vi "4Pi 4Pi Modes - Select Modes2.vi"() -> ()   [LabVIEW 2016]
uses:
  4Pi 4Pi Modes - Controls/4Pi 4Pi Modes - Mirror Modes.ctl
  <vilib>/Utility/miscctls.llb/LVPointTypeDef.ctl
  Hardware Configuration/Hardware Configuration Controls/Standard Action.ctl
  4Pi 4Pi Modes - Controls/4Pi 4Pi Modes - Standard Action.ctl
  <userlib>/BMC/BMC.lvlib
panel:
  out "error out":errorcluster
  in  "Mirror Modes":T1
  in  "Flags":string
  in  "Run":bool
  in  "Help":bool
  in  "Control mode":string(combo)="Single"
  in  "DM index":string(combo)="0"
  out "standard output":string
  out "standard error":string
  in  "Calling VI Ref":refnum<vi>
  in  "Exit":bool
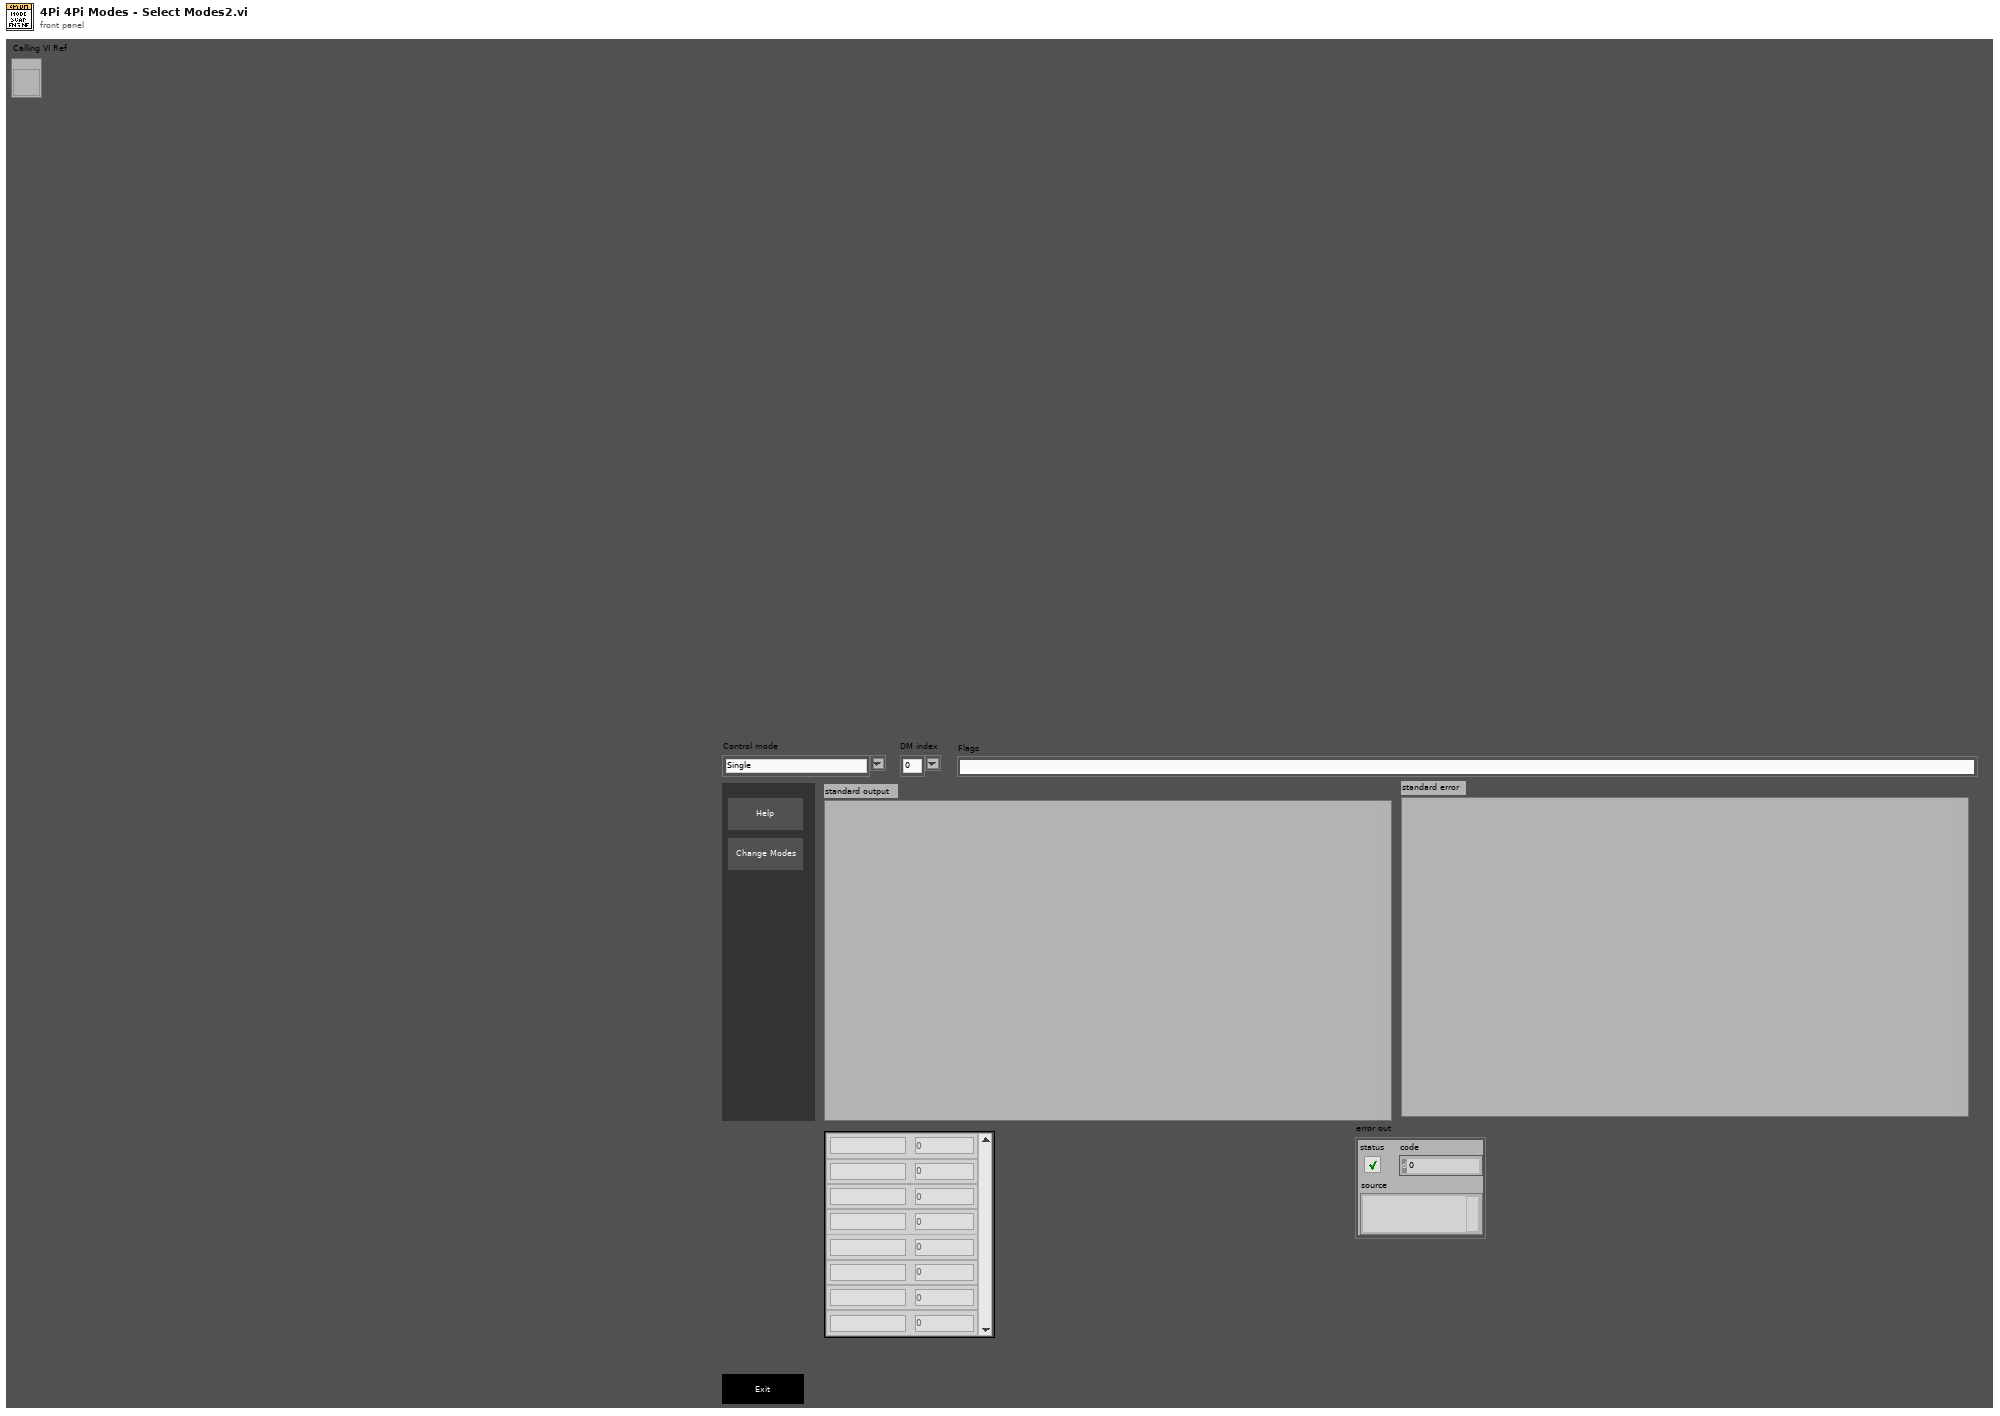
[diagram p1: front panel]
types:
  T1 = typedef "4Pi 4Pi Modes - Mirror Modes.ctl" = cluster{"Mode":string, "Amplitude":dbl}[]
  T2 = enum16{"Always On", "Always Off", "Off While Running"}
  T3 = typedef "LVPointTypeDef.ctl" = cluster{"Horizontal":i16, "Vertical":i16}
  T4 = typedef "LVRectTypeDef.ctl" = cluster{"Left":i16, "Top":i16, "Right":i16, "Bottom":i16}
  T5 = typedef "LVBoundsTypeDef.ctl" = cluster{"Width":u32, "Height":u32}
  T6 = typedef "Standard Action.ctl" = enum16{"Read", "Write"}
  T7 = typedef "4Pi 4Pi Modes - Standard Action.ctl" = enum16{"Read", "Write"}
  T8 = cluster{"type":i16, "ID":i16, "size":i32, "lutName":u64, "priv":u64}[]
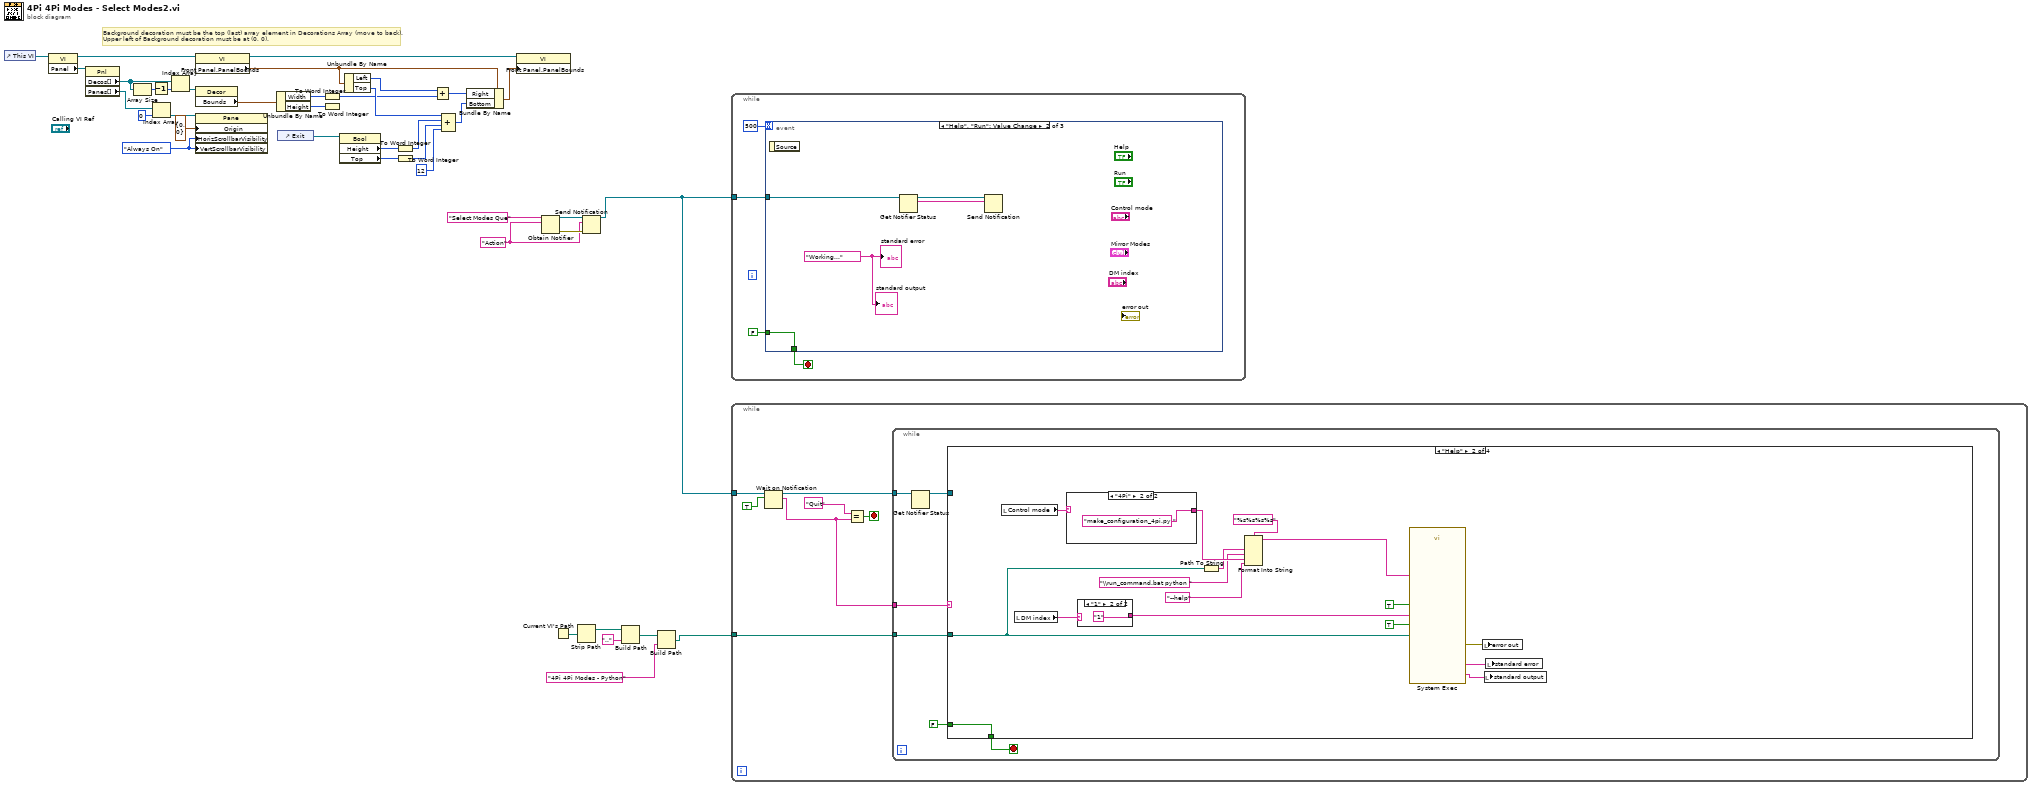
[diagram p0: block diagram]
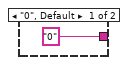
[diagram p3: hidden frame]
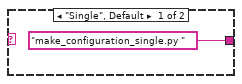
[diagram p4: hidden frame]
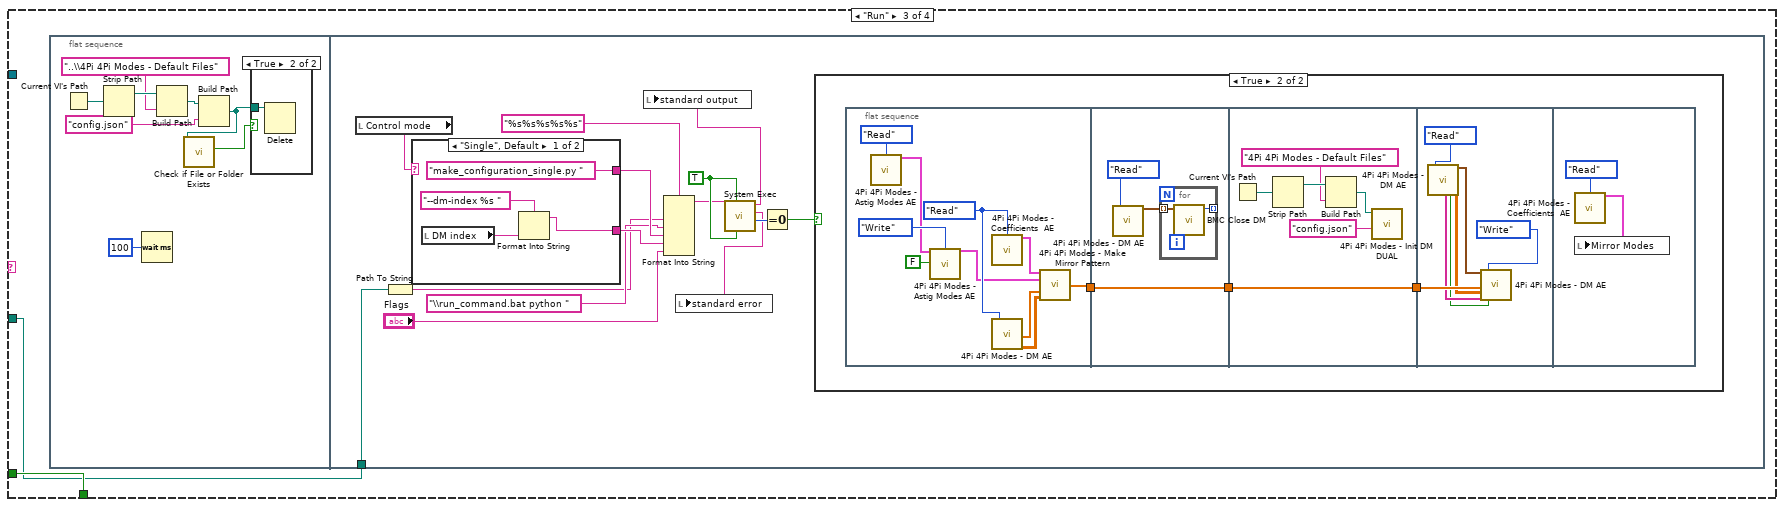
[diagram p5: hidden frame]
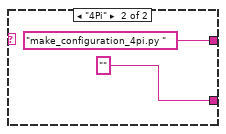
[diagram p8: hidden frame]
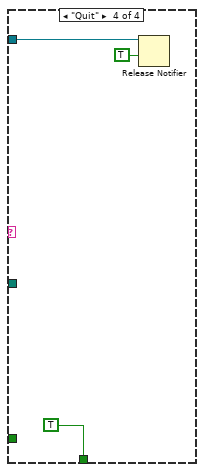
[diagram p9: hidden frame]
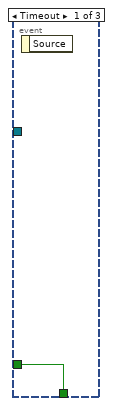
[diagram p10: hidden frame]
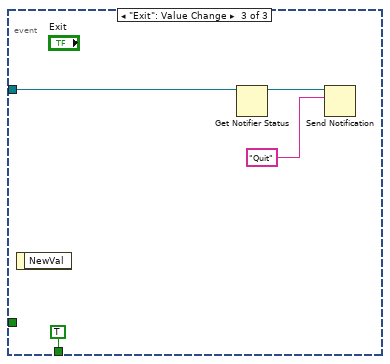
[diagram p11: hidden frame]
diagram:
  w7 = "Action" ("name (unnamed)")
  w23 = T2."Always On" ("Vertical Scrollbar Visibility")
  # "Background decoration must be the top (last) array element in Decorations Array (move to back).\nUpper left of Background decoration must be at (0, 0)."
  n1 = control-ref of="This VI"() -> (w15:refnum<vi>)
  n2 = property class="VI"(reference=w15) -> (reference out=w24:refnum<vi>, "Panel"=w16:refnum<vi>)  [unwired: 1 in, 1 out]
  n3 = property class="Pnl"(reference=w16) -> ("Decos[]"=w14:refnum<vi>[], "Panes[]"=w20:refnum<vi>[])  [unwired: 1 in, 2 out]
  n4 = Array Size(array=w14) -> (size(s)=w12:i32)
  n5 = Decrement(x=w12) -> (x-1=w13:i32)
  n6 = Index Array(array=w20, index=0) -> (element=w19:refnum<vi>)
  n7 = Index Array(array=w14, index=w13) -> (element=w22:refnum<vi>)
  n8 = property class="VI"(reference=w24) -> (reference out=w26:refnum<vi>, "Front Panel.PanelBounds"=w27:T4)  [unwired: 1 in, 1 out]
  n9 = property class="Decor"(reference=w22) -> ("Bounds"=w25:T5)  [unwired: 1 in, 2 out]
  n10 = property class="Pane"(reference=w19, "Origin"=T3 {"Horizontal"=0, "Vertical"=0}, "HorizScrollbarVisibility"=w23, "VertScrollbarVisibility"=w23) -> ()  [unwired: 1 in, 2 out]
  n11 = Unbundle By Name(w25) -> ("Width"=w30:u32, "Height"=w33:u32)
  n12 = control-ref of="Exit"() -> (w17:refnum<vi>)
  n13 = To Word Integer(number=w30) -> (16bit integer=w32:i16)
  n14 = To Word Integer(number=w33) -> ()  [unwired: 1 out]
  n15 = property class="Bool"(reference=w17) -> ("Height"=w35:u32, "Top"=w36:i32)  [unwired: 1 in, 2 out]
  n16 = Unbundle By Name(w27) -> ("Left"=w29:i16, "Top"=w40:i16)
  n17 = To Word Integer(number=w35) -> (16bit integer=w38:i16)
  n18 = To Word Integer(number=w36) -> (16bit integer=w39:i16)
  n19 = Add(x=w29, y=w32) -> (x+y=w31:i16)
  n20 = Compound Arithmetic op=ADD(w40, w38, w39, i16 12 ("y")) -> (w34:i16)
  n21 = Bundle By Name(cluster=w27, "Right"=w31, "Bottom"=w34) -> (w28:T4)
  n22 = property class="VI"(reference=w26, "Front Panel.PanelBounds"=w28) -> ()  [unwired: 1 in, 2 out]
  n23 = Obtain Notifier(name (unnamed)="Select Modes Que", notification data type=w7) -> (notifier out=w9:refnum<notifier>, error out=w10:errorcluster)  [unwired: 2 in, 1 out]
  n24 = Current VI's Path() -> (path=w5:path)
  n25 = Strip Path(path=w5) -> (stripped path=w4:path)  [unwired: 1 out]
  n26 = Send Notification(notification=w7, notifier=w9, error in (no error)=w10) -> (notifier out=w8:refnum<notifier>)  [unwired: 1 out]
  n27 = Build Path(base path=w4, name or relative path="..") -> (appended path=w2:path)
  n28 = Build Path(base path=w2, name or relative path="4Pi 4Pi Modes - Python") -> (appended path=w1:path)
  n29 = while {
    tunnel: w8 -> [w43]
    stop <- w41 stop-if-true
    n30 = event shown="[1] \"Help\", \"Run\": Value Change" {
      selector: _ -> [_ _ _]
      dyn-events: _ -> [_ _ _]
      timeout: 500 -> [_ _ _]
      tunnel: w43 -> [_ w49 w53]
      tunnel: [w45 w46 TRUE] -> w41
      tunnel: FALSE -> [w45 w46 _]
      event Timeout {
        n31 = event-data() -> ()  [unwired: 1 in, 1 out]
      }
      event "Help", "Run": Value Change {
        w47 = "Working..." ("standard error")
        n32 = event-data() -> ()  [unwired: 1 in, 1 out]
        n33 = Get Notifier Status(notifier=w49) -> (notifier out=w50:refnum<notifier>, current notification=w48:string)  [unwired: 1 in, 3 out]
        n34 = Send Notification(notification=w48, notifier=w50) -> ()  [unwired: 1 in, 2 out]
        "standard error" <- w47
        "standard output" <- w47
      }
      event "Exit": Value Change {
        n35 = event-data() -> ()  [unwired: 1 in, 1 out]
        n36 = Get Notifier Status(notifier=w53) -> (notifier out=w54:refnum<notifier>)  [unwired: 1 in, 4 out]
        n37 = Send Notification(notification="Quit", notifier=w54) -> ()  [unwired: 1 in, 2 out]
      }
    }
  }
  n38 = while {
    tunnel: w8 -> [w61]
    tunnel: w1 -> [w55]
    stop <- w58 stop-if-true
    n39 = Wait on Notification(notifier=w61, ignore previous (F)=TRUE) -> (notifier out=w59:refnum<notifier>, notification=w56:string)  [unwired: 2 in, 2 out]
    n40 = Equal?(x="Quit" ("name (unnamed)"), y=w56) -> (x = y?=w58:bool)
    n41 = while {
      tunnel: w59 -> [w66]
      tunnel: w56 -> [w63]
      tunnel: w55 -> [w62]
      stop <- w67 stop-if-true
      n42 = Get Notifier Status(notifier=w66) -> (notifier out=w65:refnum<notifier>)  [unwired: 1 in, 4 out]
      n43 = case shown="\"Help\"" w63 {
        tunnel: [w68 w70 w90 TRUE] -> w67
        tunnel: w65 -> [_ _ _ w154]
        tunnel: FALSE -> [w68 w70 w90 _]
        tunnel: w62 -> [_ w71 w89 _]
        frame "Scan Mode", Default {
        }
        frame "Help" {
          n44 = local read "Control mode"() -> (w76:string)
          n45 = local read "DM index"() -> (w83:string)
          n46 = case shown="\"4Pi\"" w76 {
            tunnel: ["make_configuration_single.py " "make_configuration_4pi.py "] -> w81
            frame "Single", Default {
            }
            frame "4Pi" {
            }
          }
          n47 = case shown="\"1\"" w83 {
            tunnel: ["0" ("name or relative path") "1" ("name or relative path")] -> w84
            frame "0", Default {
            }
            frame "1" {
            }
          }
          n48 = Path To String(path=w71) -> (string=w78:string)
          n49 = Format Into String(format string="%s%s%s%s", w78, "\\run_command.bat python " ("name or relative path"), w81, "--help" ("name or relative path")) -> (resulting string=w80:string)  [unwired: 2 in, 1 out]
          n50 = call <vilib>:"System Exec.vi"("run minimized? (F)"=TRUE, "wait until completion? (T)"=TRUE, "working directory"=w71, "standard input"=w84, "command line"=w80) -> ("error out"=w69:errorcluster, "standard error"=w74:string, "standard output"=w75:string)  [unwired: 3 in, 1 out]
          n51 = local write "error out"(w69) -> ()
          n52 = local write "standard output"(w75) -> ()
          n53 = local write "standard error"(w74) -> ()
        }
        frame "Run" {
          n54 = flat-sequence {
            tunnel: w89 -> [w103]
            frame #0 {
              n55 = Current VI's Path() -> (path=w97:path)
              n56 = Strip Path(path=w97) -> (stripped path=w98:path)  [unwired: 1 out]
              n57 = Wait (ms)(milliseconds to wait=u32 100) -> ()  [unwired: 1 out]
              n58 = Build Path(base path=w98, name or relative path="..\\4Pi 4Pi Modes - Default Files") -> (appended path=w95:path)
              n59 = Build Path(base path=w95, name or relative path="config.json") -> (appended path=w92:path)
              n60 = call <vilib>:"Check if File or Folder Exists.vi"("path"=w92) -> ("file or folder exists?"=w93:bool)  [unwired: 8 in, 2 out]
              n61 = case shown="True" w93 {
                tunnel: w92 -> [_ w99]
                frame False {
                }
                frame True {
                  n62 = Delete(path (use dialog)=w99) -> ()  [unwired: 4 in, 3 out]
                }
              }
            }
            frame #1 {
              w113 = TRUE ("run minimized? (F)")
              n63 = local read "Control mode"() -> (w104:string)
              n64 = Path To String(path=w103) -> (string=w106:string)
              n65 = case shown="\"Single\", Default" w104 {
                tunnel: ["make_configuration_single.py " "make_configuration_4pi.py "] -> w109
                tunnel: [w148 ""] -> w112
                frame "Single", Default {
                  n66 = local read "DM index"() -> (w147:string)
                  n67 = Format Into String(format string="--dm-index %s ", w147) -> (resulting string=w148:string)  [unwired: 2 in, 1 out]
                }
                frame "4Pi" {
                }
              }
              n68 = Format Into String(format string="%s%s%s%s%s", w106, "\\run_command.bat python " ("name or relative path"), w109, w112, "Flags") -> (resulting string=w108:string)  [unwired: 2 in, 1 out]
              n69 = call <vilib>:"System Exec.vi"("run minimized? (F)"=w113, "wait until completion? (T)"=w113, "command line"=w108) -> ("return code"=w110:i32, "standard error"=w101:string, "standard output"=w102:string)  [unwired: 5 in, 1 out]
              n70 = local write "standard output"(w102) -> ()
              n71 = local write "standard error"(w101) -> ()
              n72 = Equal To 0?(x=w110) -> (x = 0?=w100:bool)
              n73 = case shown="True" w100 {
                frame False {
                }
                frame True {
                  n74 = flat-sequence {
                    tunnel: [w117] -> w116
                    tunnel: w116 -> [w129]
                    tunnel: [w129] -> w115
                    tunnel: w115 -> [w132]
                    tunnel: [w132] -> w114
                    tunnel: w114 -> [w141]
                    frame #0 {
                      w123 = 4Pi_4Pi_Modes_-_Standard_Action."Read" ("Action")
                      n75 = call "4Pi 4Pi Modes - Astig Modes AE.vi"("Action"=Standard_Action."Read") -> ("Coefficients Out"=w118:cluster{"Mode":string, "Amplitude":dbl}[])  [unwired: 13 in, 1 out]
                      n76 = call "4Pi 4Pi Modes - Astig Modes AE.vi"("Coefficients In"=w118, "Action"=Standard_Action."Write", "Enabled In"=FALSE) -> ("Coefficients Out"=w121:cluster{"Mode":string, "Amplitude":dbl}[])  [unwired: 11 in, 1 out]
                      n77 = call "4Pi 4Pi Modes - Coefficients  AE.vi"("Action"=w123) -> ("Coefficients Out"=w122:cluster{"Mode":string, "Amplitude":dbl}[])  [unwired: 14 in]
                      n78 = call "4Pi 4Pi Modes - DM AE.vi"("Action"=w123) -> ("Flats Out"=w120:dbl[], "Control Matrix Out"=w119:dbl[][])  [unwired: 14 in, 3 out]
                      n79 = call "4Pi 4Pi Modes - Make Mirror Pattern.vi"("Coefficients"=w122, "Astig Coeffs"=w121, "Flats"=w120, "Control Matrix"=w119) -> ("Pixel Value U (-1 to 1)"=w117:dbl[])  [unwired: 10 in, 1 out]
                    }
                    frame #1 {
                      n80 = call "4Pi 4Pi Modes - DM AE.vi"("Action"=4Pi_4Pi_Modes_-_Standard_Action."Read") -> ("DM Handles Out"=w127:T8)  [unwired: 14 in, 4 out]
                      n81 = for {
                        tunnel: w127 -> [w131] mode=indexing
                        tunnel: [w130] -> _ mode=indexing
                        n82 = call <userlib>:"BMC Close DM.vi"("dmHandle"=w131) -> ("function return"=w130:i32)  [unwired: 9 in, 1 out]
                      }
                    }
                    frame #2 {
                      n83 = Current VI's Path() -> (path=w134:path)
                      n84 = Strip Path(path=w134) -> (stripped path=w135:path)  [unwired: 1 out]
                      n85 = Build Path(base path=w135, name or relative path="4Pi 4Pi Modes - Default Files") -> (appended path=w137:path)
                      n86 = call "4Pi 4Pi Modes - Init DM DUAL.vi"("Config File"="config.json" ("name or relative path"), "Base File Path"=w137) -> ()  [unwired: 8 in, 2 out]
                    }
                    frame #3 {
                      n87 = call "4Pi 4Pi Modes - DM AE.vi"("Action"=4Pi_4Pi_Modes_-_Standard_Action."Read") -> ("Serials Out"=w139:string[], "No hardware Out"=w138:bool, "DM Handles Out"=w142:T8, "Control Matrix Out"=w140:dbl[][])  [unwired: 14 in, 1 out]
                      n88 = call "4Pi 4Pi Modes - DM AE.vi"("DM Handles"=w142, "Flats"=w141, "Control Matrix"=w140, "Serials"=w139, "Action"=4Pi_4Pi_Modes_-_Standard_Action."Write", "No hardware"=w138) -> ()  [unwired: 9 in, 5 out]
                    }
                    frame #4 {
                      n89 = call "4Pi 4Pi Modes - Coefficients  AE.vi"("Action"=4Pi_4Pi_Modes_-_Standard_Action."Read") -> ("Coefficients Out"=w145:cluster{"Mode":string, "Amplitude":dbl}[])  [unwired: 14 in]
                      n90 = local write "Mirror Modes"(w145) -> ()
                    }
                  }
                }
              }
            }
          }
        }
        frame "Quit" {
          n91 = Release Notifier(notifier=w154, force destroy? (F)=TRUE) -> ()  [unwired: 1 in, 3 out]
        }
      }
    }
  }
